vi "GetAllPaths.vi"(0 "LocalName":string) -> (1 "Hard Path":path, 2 "Top Level":path, 3 "User Documents":path)   [LabVIEW 2014]
doc: "Gets the paths for LVROS, the servers, _BlankServer, and the Master Console"
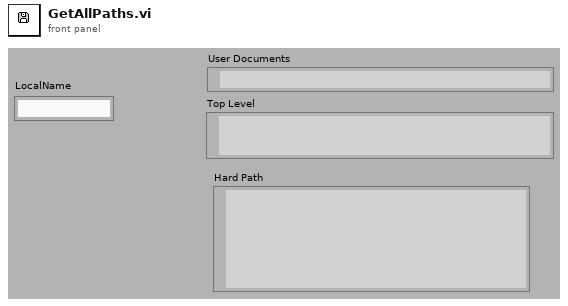
[diagram p1: front panel]
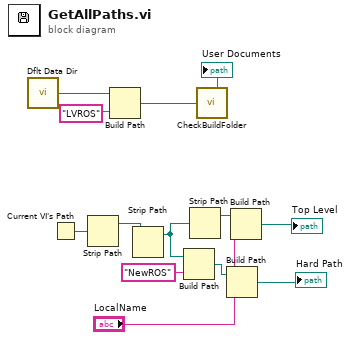
[diagram p0: block diagram]
diagram:
  n1 = call <vilib>:"Dflt Data Dir.vi"() -> ("App:Default Data Directory"=w10:path)
  n2 = Current VI's Path() -> (path=w12:path)
  n3 = Strip Path(path=w12) -> (stripped path=w8:path)  [unwired: 1 out]
  n4 = Build Path(base path=w10, name or relative path="LVROS") -> (appended path=w9:path)
  "User Documents" <- w9
  n5 = Strip Path(path=w8) -> (stripped path=w4:path)  [unwired: 1 out]
  n6 = Build Path(base path=w4, name or relative path="NewROS") -> (appended path=w7:path)
  n7 = Strip Path(path=w4) -> (stripped path=w3:path)  [unwired: 1 out]
  n8 = call "CheckBuildFolder.vi"("appended path"=w9) -> ()  [unwired: 1 in]
  n9 = Build Path(base path=w7, name or relative path="LocalName") -> (appended path=→"Hard Path":path)
  n10 = Build Path(base path=w3, name or relative path="LocalName") -> (appended path=→"Top Level":path)
